vi "test Update Alias Endpoint.vi"(8 "error in (no error)":errorcluster, 11 "TestCase in":refnum<class "Routing and Faulting Aliases Unit Tests.lvclass">) -> (0 "error out":errorcluster, 3 "TestCase out":refnum<class "Routing and Faulting Aliases Unit Tests.lvclass">)   [LabVIEW 2020, in "Routing and Faulting Aliases Unit Tests.lvclass"]
uses:
  Routing and Faulting Aliases Unit Tests.lvclass
  System Explorer/Alias.ctl
  System Explorer/Endpoint.ctl
  Shared/Alias Mapping.ctl
  Shared/Alias Endpoint.ctl
  Routing and Faulting Aliases Unit Tests.lvclass/Routing and Faulting Aliases Unit Tests.ctl
  <vilib>/addons/_JKI Toolkits/VI Tester/TestCase.llb/TestCase.lvclass
  System Explorer/Routing and Faulting System Explorer.lvlib
  Scripting/Routing and Faulting Scripting.lvlib
  Shared/Routing and Faulting Shared.lvlib
  C:/Program Files (x86)/National Instruments/LabVIEW 2020/vi.lib/addons/_JKI Toolkits/VI Tester/TestCase.llb/TestCase.lvclass
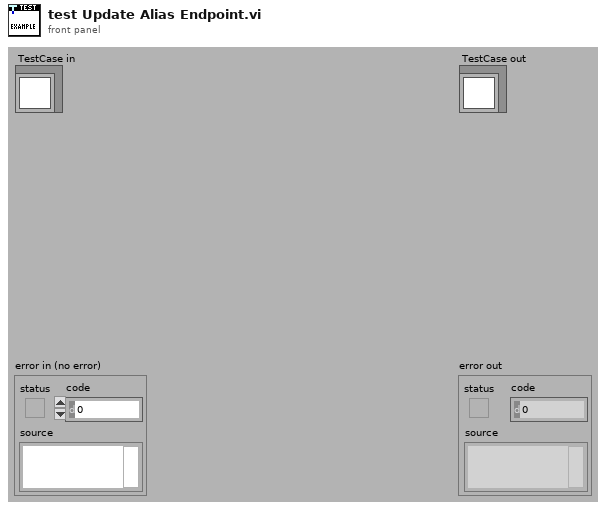
[diagram p1: front panel]
types:
  T1 = typedef "Routing and Faulting System Explorer.lvlib/Endpoint.ctl" = string
  T2 = typedef "Routing and Faulting Shared.lvlib/Alias Endpoint.ctl" = cluster{"Module Path":string, "Endpoint":string}
  T3 = typedef "Routing and Faulting Shared.lvlib/Alias Mapping.ctl" = cluster{"Alias":string, "Endpoint":T2}
  T4 = typedef "Routing and Faulting System Explorer.lvlib/Alias.ctl" = cluster{"Endpoint":T1, "Alias":string, "Remove":bool}
  T5 = typedef "Custom Device API.lvlib/Custom Device Item Ref.ctl" = u64
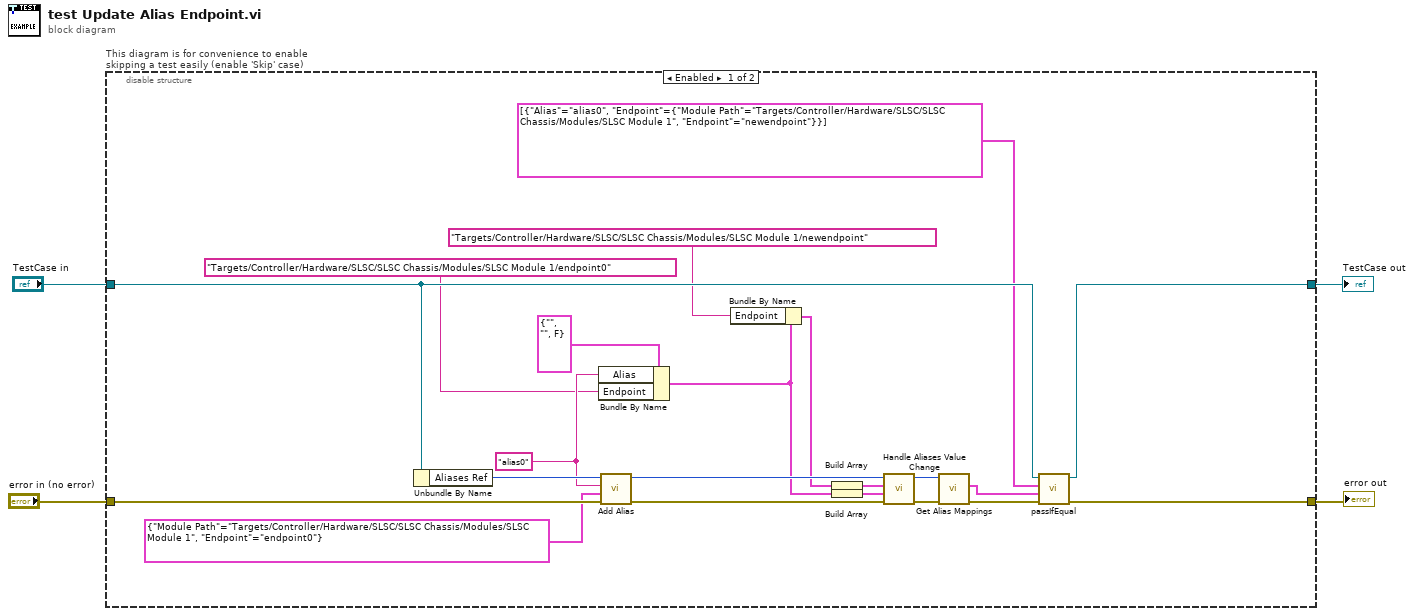
[diagram p0: block diagram]
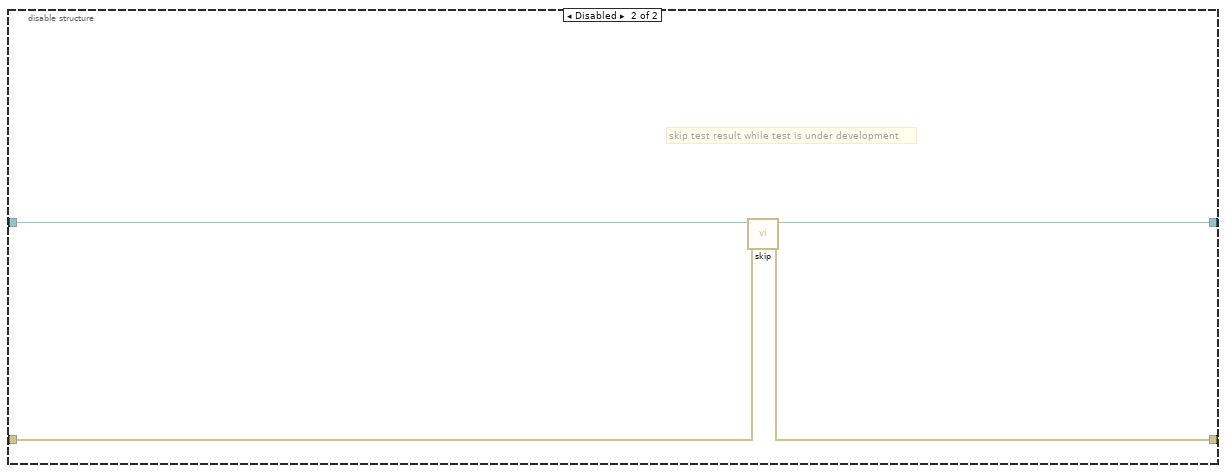
[diagram p2: hidden frame]
diagram:
  n1 = disable-structure "This diagram is for convenience to enable skipping a test easily (enable 'Skip' case)" shown="Enabled" {
    disable-tunnel: "TestCase in" -> [w20 w29]
    disable-tunnel: [w19 w27] -> w1
    disable-tunnel: [w22 w28] -> w3
    disable-tunnel: "error in (no error)" -> [w17 w26]
    frame Enabled {
      w13 = "alias0" ("Alias")
      n2 = Unbundle By Name(w20) -> ("Aliases Ref"=w18:T5)
      n3 = Bundle By Name(cluster=T4 {"Endpoint"="", "Alias"="", "Remove"=FALSE} ("Alias"), "Alias"=w13, "Endpoint"=T1 "Targets/Controller/Hardware/SLSC/SLSC Chassis/Modules/SLSC Module 1/endpoint0") -> (w11:T4)
      n4 = call "Add Alias.vi"("error in"=w17, "endpoint"=T2 {"Module Path"="Targets/Controller/Hardware/SLSC/SLSC Chassis/Modules/SLSC Module 1", "Endpoint"="endpoint0"} ("Endpoint"), "alias"=w13, "endpoint aliases in"=w18) -> ("error out"=w15:errorcluster, "endpoint aliases out"=w16:T5)  [unwired: 6 in]
      n5 = Bundle By Name(cluster=w11, "Endpoint"=T1 "Targets/Controller/Hardware/SLSC/SLSC Chassis/Modules/SLSC Module 1/newendpoint") -> (w10:T4)
      n6 = Build Array(w10) -> (w8:T4[])
      n7 = Build Array(w11) -> (w9:T4[])
      n8 = call "Handle Aliases Value Change.vi"("error in (no error)"=w15, "OldVal"=w9, "NewVal"=w8, "Aliases Ref in"=w16) -> ("error out"=w25:errorcluster, "Aliases Ref out"=w24:T5)  [unwired: 4 in, 2 out]
      n9 = call "Get Alias Mappings.vi"("error in"=w25, "endpoint aliases in"=w24) -> ("error out"=w23:errorcluster, "alias mappings"=w21:T3[])  [unwired: 7 in, 1 out]
      n10 = call-dynamic "passIfEqual.vi"("error in (no error)"=w23, "y"=w21, "x"=T3[] [{"Alias"="alias0", "Endpoint"={"Module Path"="Targets/Controller/Hardware/SLSC/SLSC Chassis/Modules/SLSC Module 1", "Endpoint"="newendpoint"}}] ("Alias Mappings"), "TestCase in"=w20) -> ("error out"=w22:errorcluster, "TestCase out"=w19:refnum<class "Routing and Faulting Aliases Unit Tests.lvclass">)  [unwired: 6 in]
    }
    frame Disabled {
      # "skip test result while test is under development"
      n11 = call <vilib>:"skip.vi"("error in (no error)"=w26, "TestCase in"=w29) -> ("error out"=w28:errorcluster, "TestCase out"=w27:refnum<class "Routing and Faulting Aliases Unit Tests.lvclass">)  [unwired: 8 in]
    }
  }
  "error out" <- w3
  "TestCase out" <- w1
